vi "Mediciones.vi"() -> ()   [LabVIEW 2017]
panel:
  in  "Alto":dbl
  in  "Ancho":dbl
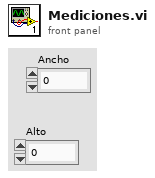
[diagram p1: front panel]
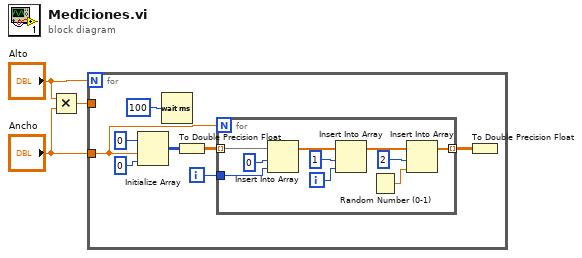
[diagram p0: block diagram]
diagram:
  n1 = Multiply(x="Alto", y="Ancho") -> (x*y=w3:dbl)
  n2 = for {
    N: "Alto" -> [_]
    tunnel: "Ancho" -> [w6]
    tunnel: w3 -> [_]
    i -> [w4]
    n3 = Initialize Array(0, w6, 0) -> (w8:i32[][])
    n4 = Wait (ms)(milliseconds to wait=100) -> ()  [unwired: 1 out]
    n5 = To Double Precision Float(number=w8) -> (double precision float=w9:dbl[][])
    n6 = for {
      N: w6 -> [_]
      tunnel: w9 -> [w13] mode=indexing
      tunnel: [w16] -> w7 mode=indexing
      tunnel: w4 -> [w14]
      i -> [w21]
      n7 = Insert Into Array(array=w13, index=0, new element=w14) -> (w12:dbl[])
      n8 = Insert Into Array(array=w12, index=1, new element=w21) -> (w19:dbl[])
      n9 = Random Number (0-1)() -> (number: 0 to 1=w17:dbl)
      n10 = Insert Into Array(array=w19, index=2, new element=w17) -> (w16:dbl[])
    }
    n11 = To Double Precision Float(number=w7) -> ()  [unwired: 1 out]
  }
